vi "Contiguous Value Search.vi"(6 "Sorted Default Value (in)":string[](array[string])=["1.0", "2.0", "3.0", "4.0", "5.0", "6.0"], 7 "Tx?":bool, 8 "Sorted Name (in)":string[](array[string])=["cat", "dog", "bird", "snake", "donkey", "rat"], 10 "Sorted Array (in)":i32[](array[numeric])=[4, 5, 8, 9, 67, 68], 11 "String (in)":string) -> (3 "String (out)":string)   [LabVIEW 2017]
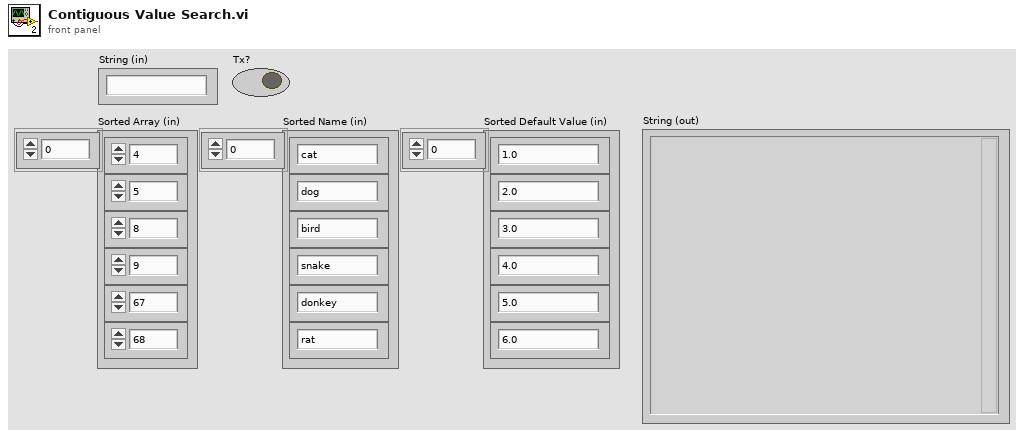
[diagram p1: front panel]
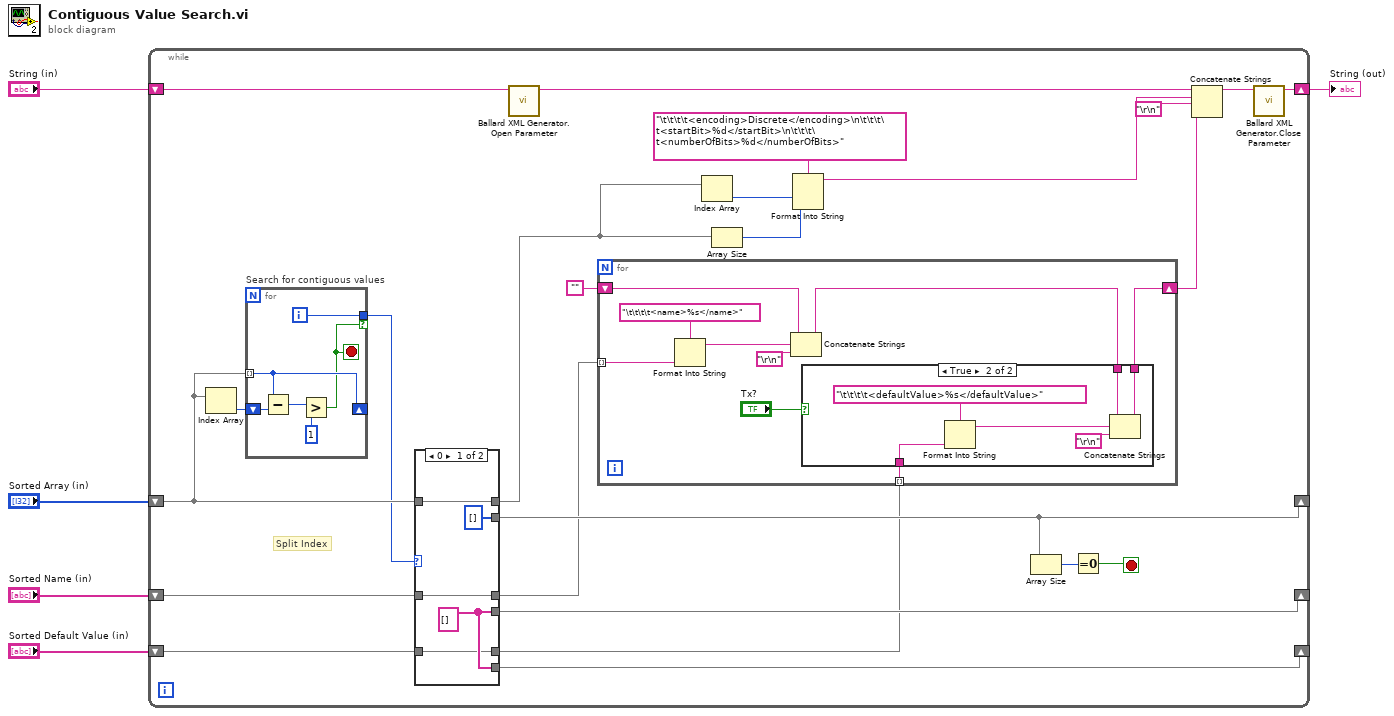
[diagram p0: block diagram]
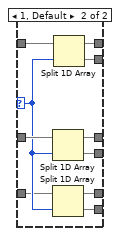
[diagram p3: hidden frame]
diagram:
  n1 = while {
    shift-right: [w26] -> _
    shift-left: "Sorted Name (in)" -> [w28]
    shift-right: [w25] -> _
    shift-left: "Sorted Array (in)" -> [w27]
    shift-right: [w14] -> w2
    shift-left: "String (in)" -> [w12]
    shift-right: [w8] -> _
    shift-left: "Sorted Default Value (in)" -> [w9]
    stop <- w22 stop-if-true
    # "Split Index"
    n2 = Index Array(array=w27) -> (element=w29:i32)  [unwired: 1 in]
    n3 = for "Search for contiguous values" {
      tunnel: w27 -> [w63] mode=indexing
      shift-right: [w63] -> _
      shift-left: w29 -> [w66]
      tunnel: [w62] -> w24 if=w61
      i -> [w62]
      stop <- w61 stop-if-true
      n4 = Subtract(x=w63, y=w66) -> (x-y=w65:i32)
      n5 = Greater?(x=w65, y=1) -> (0:w61:bool)
    }
    n6 = case shown="0" w24 {
      selector: w24 -> [_ w54]
      tunnel: w28 -> [w49 w60]
      tunnel: [w49 w59] -> w21
      tunnel: w27 -> [w50 w58]
      tunnel: [w50 w57] -> w11
      tunnel: [w47 w56] -> w26
      tunnel: [i32[] [] w55] -> w25
      tunnel: w9 -> [w46 w53]
      tunnel: [w47 w52] -> w8
      tunnel: [w46 w51] -> w7
      frame 0 {
        w47 = string[] []
      }
      frame 1, Default {
        n7 = Split 1D Array(array=w60, index=w54) -> (first subarray=w59:string[], second subarray=w56:string[])
        n8 = Split 1D Array(array=w53, index=w54) -> (first subarray=w51:string[], second subarray=w52:string[])
        n9 = Split 1D Array(array=w58, index=w54) -> (first subarray=w57:i32[], second subarray=w55:i32[])
      }
    }
    n10 = call "Ballard XML Generator.Open Parameter.vi"("string in"=w12) -> ("string out"=w16:string)  [unwired: 10 in]
    n11 = for {
      tunnel: w21 -> [w35] mode=indexing
      shift-right: [w32] -> w6
      shift-left: "" -> [w34]
      tunnel: w7 -> [w31] mode=indexing
      n12 = Format Into String(format string="\t\t\t\t<name>%s</name>", w35) -> (resulting string=w38:string)  [unwired: 2 in, 1 out]
      n13 = Concatenate Strings(w34, w38, "\r\n") -> (w33:string)
      n14 = case shown="True" "Tx?" {
        tunnel: w33 -> [w39 w42]
        tunnel: [w39 w41] -> w32
        tunnel: w31 -> [_ w40]
        frame False {
        }
        frame True {
          n15 = Format Into String(format string="\t\t\t\t<defaultValue>%s</defaultValue>", w40) -> (resulting string=w45:string)  [unwired: 2 in, 1 out]
          n16 = Concatenate Strings(w42, w45, "\r\n") -> (w41:string)
        }
      }
    }
    n17 = Index Array(array=w11) -> (element=w19:i32)  [unwired: 1 in]
    n18 = Array Size(array=w11) -> (size(s)=w18:i32)
    n19 = Format Into String(format string="\t\t\t\t<encoding>Discrete</encoding>\n\t\t\t\t<startBit>%d</startBit>\n\t\t\t\t<numberOfBits>%d</numberOfBits>", w19, w18) -> (resulting string=w13:string)  [unwired: 2 in, 1 out]
    n20 = Array Size(array=w25) -> (size(s)=w23:i32)
    n21 = Equal To 0?(x=w23) -> (x = 0?=w22:bool)
    n22 = Concatenate Strings(w16, w13, "\r\n", w6) -> (w15:string)
    n23 = call "Ballard XML Generator.Close Parameter.vi"("string in"=w15) -> ("string out"=w14:string)  [unwired: 10 in]
  }
  "String (out)" <- w2
